vi "RemoveABus.vi"(7 "Remove All (F)":bool, 8 "ErrorArray In":errorcluster[](array[cluster]), 10 "BusNum":u8) -> (0 "ErrorArray Out":errorcluster[](array[cluster]), 3 "Bus Out":refnum<class "Bus.lvclass">)   [LabVIEW 2014]
uses:
  Bus.lvclass
  Bus.lvclass/Bus.ctl
  Accessors/Write AppModuleID.vi
  Accessors/Write OutputToFileModuleID.vi
  <vilib>/Utility/error.llb/Error Cluster From Error Code.vi
  <vilib>/ErrorRing/Error Ring.xnode
  <userlib>/NIST/NISTErrorLib/NISTErrorLib.lvlib
  Framework.lvlib
  Bus_class.lvlib
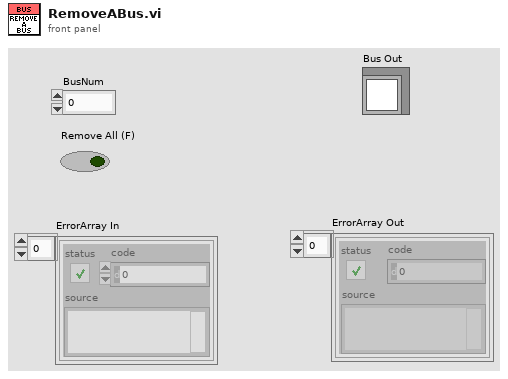
[diagram p1: front panel]
types:
  T1 = typedef "Framework.lvlib/clFrameworkData.ctl" = cluster{"EvtINIFilePaths":path[], "BusClassInstances":refnum<class "Bus.lvclass">[], "PmuImpairINIFilePaths":path[], "FlagImpairINIFilePaths":path[], "NetImpairINIFilePaths":path[], "OutputToFileINIFilePaths":path[], "AppINIFilePaths":path[], "AppModuleID":i32, "OutputToFileID":i32}
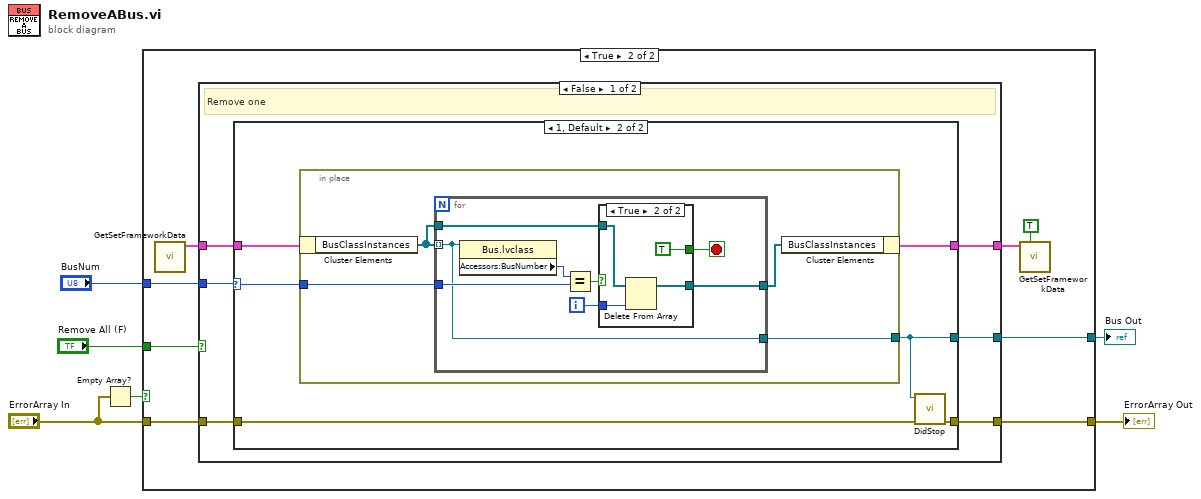
[diagram p0: block diagram]
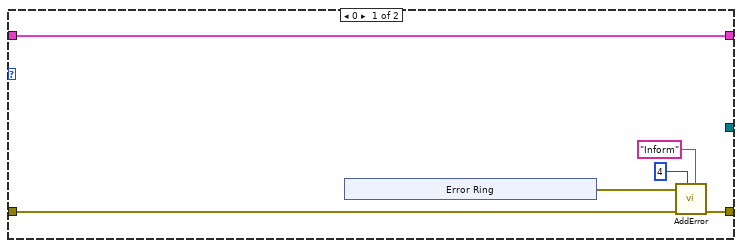
[diagram p3: hidden frame]
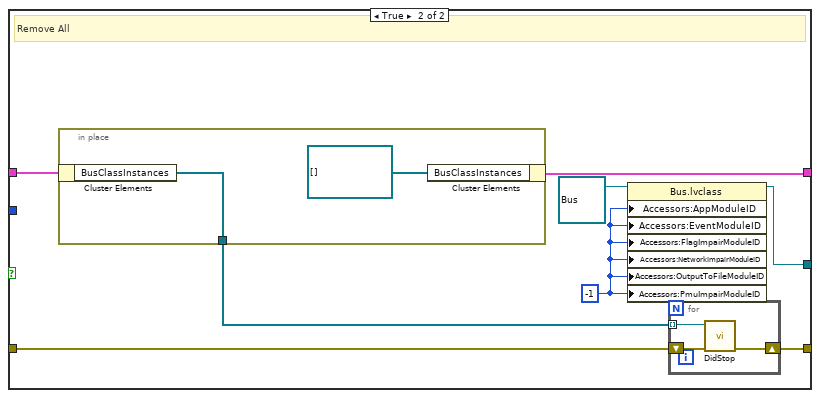
[diagram p5: hidden frame]
diagram:
  n1 = Empty Array?(array="ErrorArray In") -> (empty?=w5:bool)
  n2 = case shown="True" w5 {
    tunnel: "ErrorArray In" -> [w7 w15]
    tunnel: [w7 w14] -> w4
    tunnel: "Remove All (F)" -> [_ w13]
    tunnel: "BusNum" -> [_ w12]
    tunnel: [_ w11] -> w1
    frame False {
    }
    frame True {
      n3 = call "GetSetFrameworkData.vi"() -> ("clFrameworkData Out"=w10:T1)  [unwired: 11 in]
      n4 = case shown="False" w13 {
        tunnel: w15 -> [w21 w62]
        tunnel: [w20 w60] -> w14
        tunnel: w12 -> [w19 _]
        tunnel: [w18 w56] -> w11
        tunnel: w10 -> [w17 w63]
        tunnel: [w16 w59] -> w8
        frame False {
          # "Remove one"
          n5 = case shown="1, Default" w19 {
            selector: w19 -> [_ w38]
            tunnel: w21 -> [w23 w35]
            tunnel: [w27 w34] -> w20
            tunnel: [_ w33] -> w18
            tunnel: w17 -> [w22 w37]
            tunnel: [w22 w36] -> w16
            frame 0 {
              n6 = xnode "Error Ring"() -> ("error out"=w24:errorcluster)
              n7 = call <userlib>:"AddError.vi"("Severity"="Inform", "Priority"=u8 4, "ErrorArray"=w23, "error in (no error)"=w24) -> ("ErrorArray"=w27:errorcluster[])  [unwired: 6 in, 1 out]
            }
            frame 1, Default {
              n8 = in-place {
                in-place-border: w38 -> [w42]
                in-place-border: [w39] -> w33
                n9 = in-place-cluster #1(w37) -> ("BusClassInstances"=w41:refnum<class "Bus.lvclass">[])
                n10 = for {
                  tunnel: w41 -> [w44] mode=indexing
                  tunnel: w42 -> [w50]
                  tunnel: w41 -> [w46]
                  tunnel: [w45] -> w40
                  tunnel: [w44] -> w39
                  i -> [w47]
                  stop <- w43 stop-if-true
                  n11 = property class="Bus.lvclass"(reference=w44) -> ("Accessors:BusNumber"=w49:u8)  [unwired: 1 in, 2 out]
                  n12 = Equal?(x=w49, y=w50) -> (x = y?=w48:bool)
                  n13 = case shown="True" w48 {
                    tunnel: w47 -> [_ w55]
                    tunnel: w46 -> [w51 w54]
                    tunnel: [w51 w53] -> w45
                    tunnel: [_ TRUE] -> w43
                    frame False {
                    }
                    frame True {
                      n14 = Delete From Array(array=w54, index=w55) -> (array with subset deleted=w53:refnum<class "Bus.lvclass">[])  [unwired: 1 in, 1 out]
                    }
                  }
                }
                n15 = in-place-cluster #1("BusClassInstances"=w40) -> (w36:T1)
              }
              n16 = call "DidStop.vi"("ErrorArray"=w35, "Bus"=w33) -> ("ErrorArray"=w34:errorcluster[])  [unwired: 8 in, 1 out]
            }
          }
        }
        frame True {
          w57 = -1 ("PmuImpairModuleID")
          # "Remove All"
          n17 = in-place {
            in-place-border: [w67] -> w61
            n18 = in-place-cluster #2(w63) -> ("BusClassInstances"=w67:refnum<class "Bus.lvclass">[])
            n19 = in-place-cluster #2("BusClassInstances"=refnum<class "Bus.lvclass">[] []) -> (w59:T1)
          }
          n20 = property class="Bus.lvclass"(reference=refnum<class "Bus.lvclass"> refnum ("Bus_class.lvlib:Bus.lvclass"), "Accessors:AppModuleID"=w57, "Accessors:EventModuleID"=w57, "Accessors:FlagImpairModuleID"=w57, "Accessors:NetworkImpairModuleID"=w57, "Accessors:OutputToFileModuleID"=w57, "Accessors:PmuImpairModuleID"=w57) -> (reference out=w56:refnum<class "Bus.lvclass">)  [unwired: 1 in, 1 out]
          n21 = for {
            shift-right: [w65] -> w60
            shift-left: w62 -> [w66]
            tunnel: w61 -> [w64] mode=indexing
            n22 = call "DidStop.vi"("ErrorArray"=w66, "Bus"=w64) -> ("ErrorArray"=w65:errorcluster[])  [unwired: 8 in, 1 out]
          }
        }
      }
      n23 = call "GetSetFrameworkData.vi"("Set (F)"=TRUE, "clFrameworkData In"=w8) -> ()  [unwired: 9 in, 1 out]
    }
  }
  "ErrorArray Out" <- w4
  "Bus Out" <- w1
